vi "Set Units.vi"(2 "Assign  loss unit according to the chart on the right":dbl=1.0, 3 "VISA resource name":refnum<visa-resource-name>="GPIB12::28::INSTR") -> (0 "Read out result":string="UC= 9456.092   PF L= 658.76     NS V=0.10   V\r\n", 1 "Send string":string="UNITS 1;\nSHOW UN")   [LabVIEW 2016, in "AH2500A.lvclass"]
uses:
  SMOs/AH2500A/AH2500A.lvclass
panel:
  in  "byte count":u32=128
  out "error out":errorcluster {"code" format="%.0x"}
  in  "error in":errorcluster {"code" format="%.0x"}
  # "Set the lossunit"
  # "Default setting is 1"
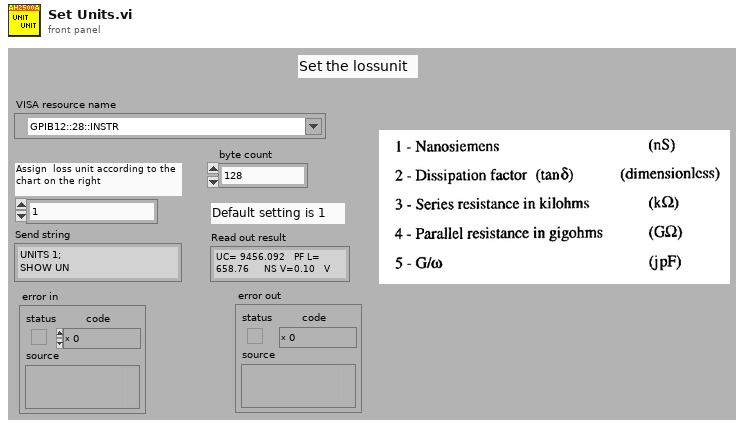
[diagram p1: front panel]
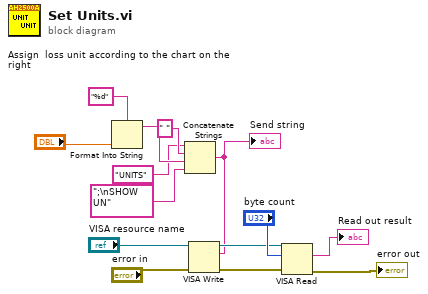
[diagram p0: block diagram]
diagram:
  n1 = Format Into String(format string="%d", "Assign  loss unit according to the chart on the right") -> (resulting string=w10:string)  [unwired: 2 in, 1 out]
  n2 = Concatenate Strings("UNITS" ("string"), " " ("string"), w10, ";\nSHOW UN" ("format string")) -> (w3:string)
  "Send string" <- w3
  n3 = VISA Write(VISA resource name="VISA resource name", write buffer=w3, error in (no error)="error in") -> (VISA resource name out=w6:refnum<visa-resource-name>, error out=w5:errorcluster)  [unwired: 1 out]
  n4 = VISA Read(VISA resource name=w6, byte count="byte count", error in (no error)=w5) -> (read buffer=→"Read out result":string, error out=→"error out":errorcluster)  [unwired: 2 out]
